vi "DRAW FP TURNOS IN UI.vi"(8 "error in (no error)":errorcluster, 11 "Turnos in":refnum<class "Turnos.lvclass">) -> (0 "error out":errorcluster, 3 "Turnos out":refnum<class "Turnos.lvclass">)   [LabVIEW 2020, in "Turnos.lvlib" / "Turnos.lvclass"]
uses:
  Turnos.lvclass
  Turnos.lvclass/Turnos.ctl
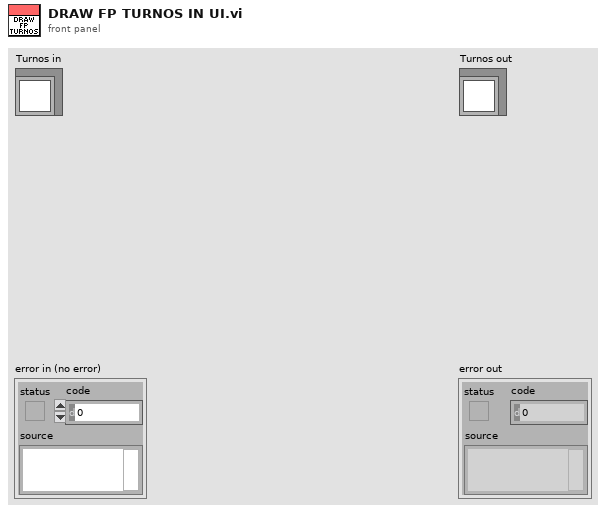
[diagram p1: front panel]
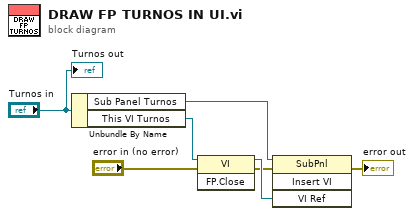
[diagram p0: block diagram]
diagram:
  n1 = Unbundle By Name("Turnos in") -> ("Sub Panel Turnos"=w1:refnum<vi>, "This VI Turnos"=w3:refnum<vi>)
  n2 = invoke class="VI" method="FP.Close"(reference=w3, error in="error in (no error)") -> (reference out=w4:refnum<vi>, error out=w2:errorcluster)  [unwired: 1 in, 1 out]
  n3 = invoke class="SubPnl" method="Insert VI"(reference=w1, error in=w2, "VI Ref"=w4) -> (error out=→"error out":errorcluster)  [unwired: 1 in, 3 out]
  "Turnos out" <- "Turnos in"
